vi "HEWH Standard MW100 Data.vi"(4 "Flow Selector":T1, 7 "Emerson Flow Meter Data Output":T2, 8 "Error In":errorcluster, 11 "MW100 Data Cluster":T3) -> (0 "Error Out":errorcluster, 2 "Hot Side Emerson Flow Meter Data":T2, 3 "Standard MW100 Data":string[][](array[string])=[["T1", "0.000"], ["T2", "0.000"], ["T3", "0.000"], ["T4", "0.000"], ["T5", "0.000"], ["T6", "0.000"], ["T7", "0.000"], ["T8", "0.000"], ["T9", "0.000"], ["T10", "0.000"], ["TC Tree Average", "0.000"], ["TC Down", "0.000"], ["RTD IN", "0.000"], ["RTD Out", "0.000"], ["RTD Ambient", "0.000"], ["Totalized Flow (Linear Link) - Calculated (Gallons)", "0.000"], ["Flow Rate (Linear Link) - Calculated (GPM)", "0.000"], ["Pressure - HI1", "0.000"], ["Pressure - HI2", "0.000"], ["Pressure - LOW", "0.000"], ["Pressure - PIN", "0.000"]])   [LabVIEW 2020]
uses:
  Type Definitions/HEWH MW100 Data Cluster.ctl
  Drivers/Emerson 5700 Transmitter/Type Definitions/Emerson 5700 Data.ctl
  Type Definitions/Flow Meter Selector.ctl
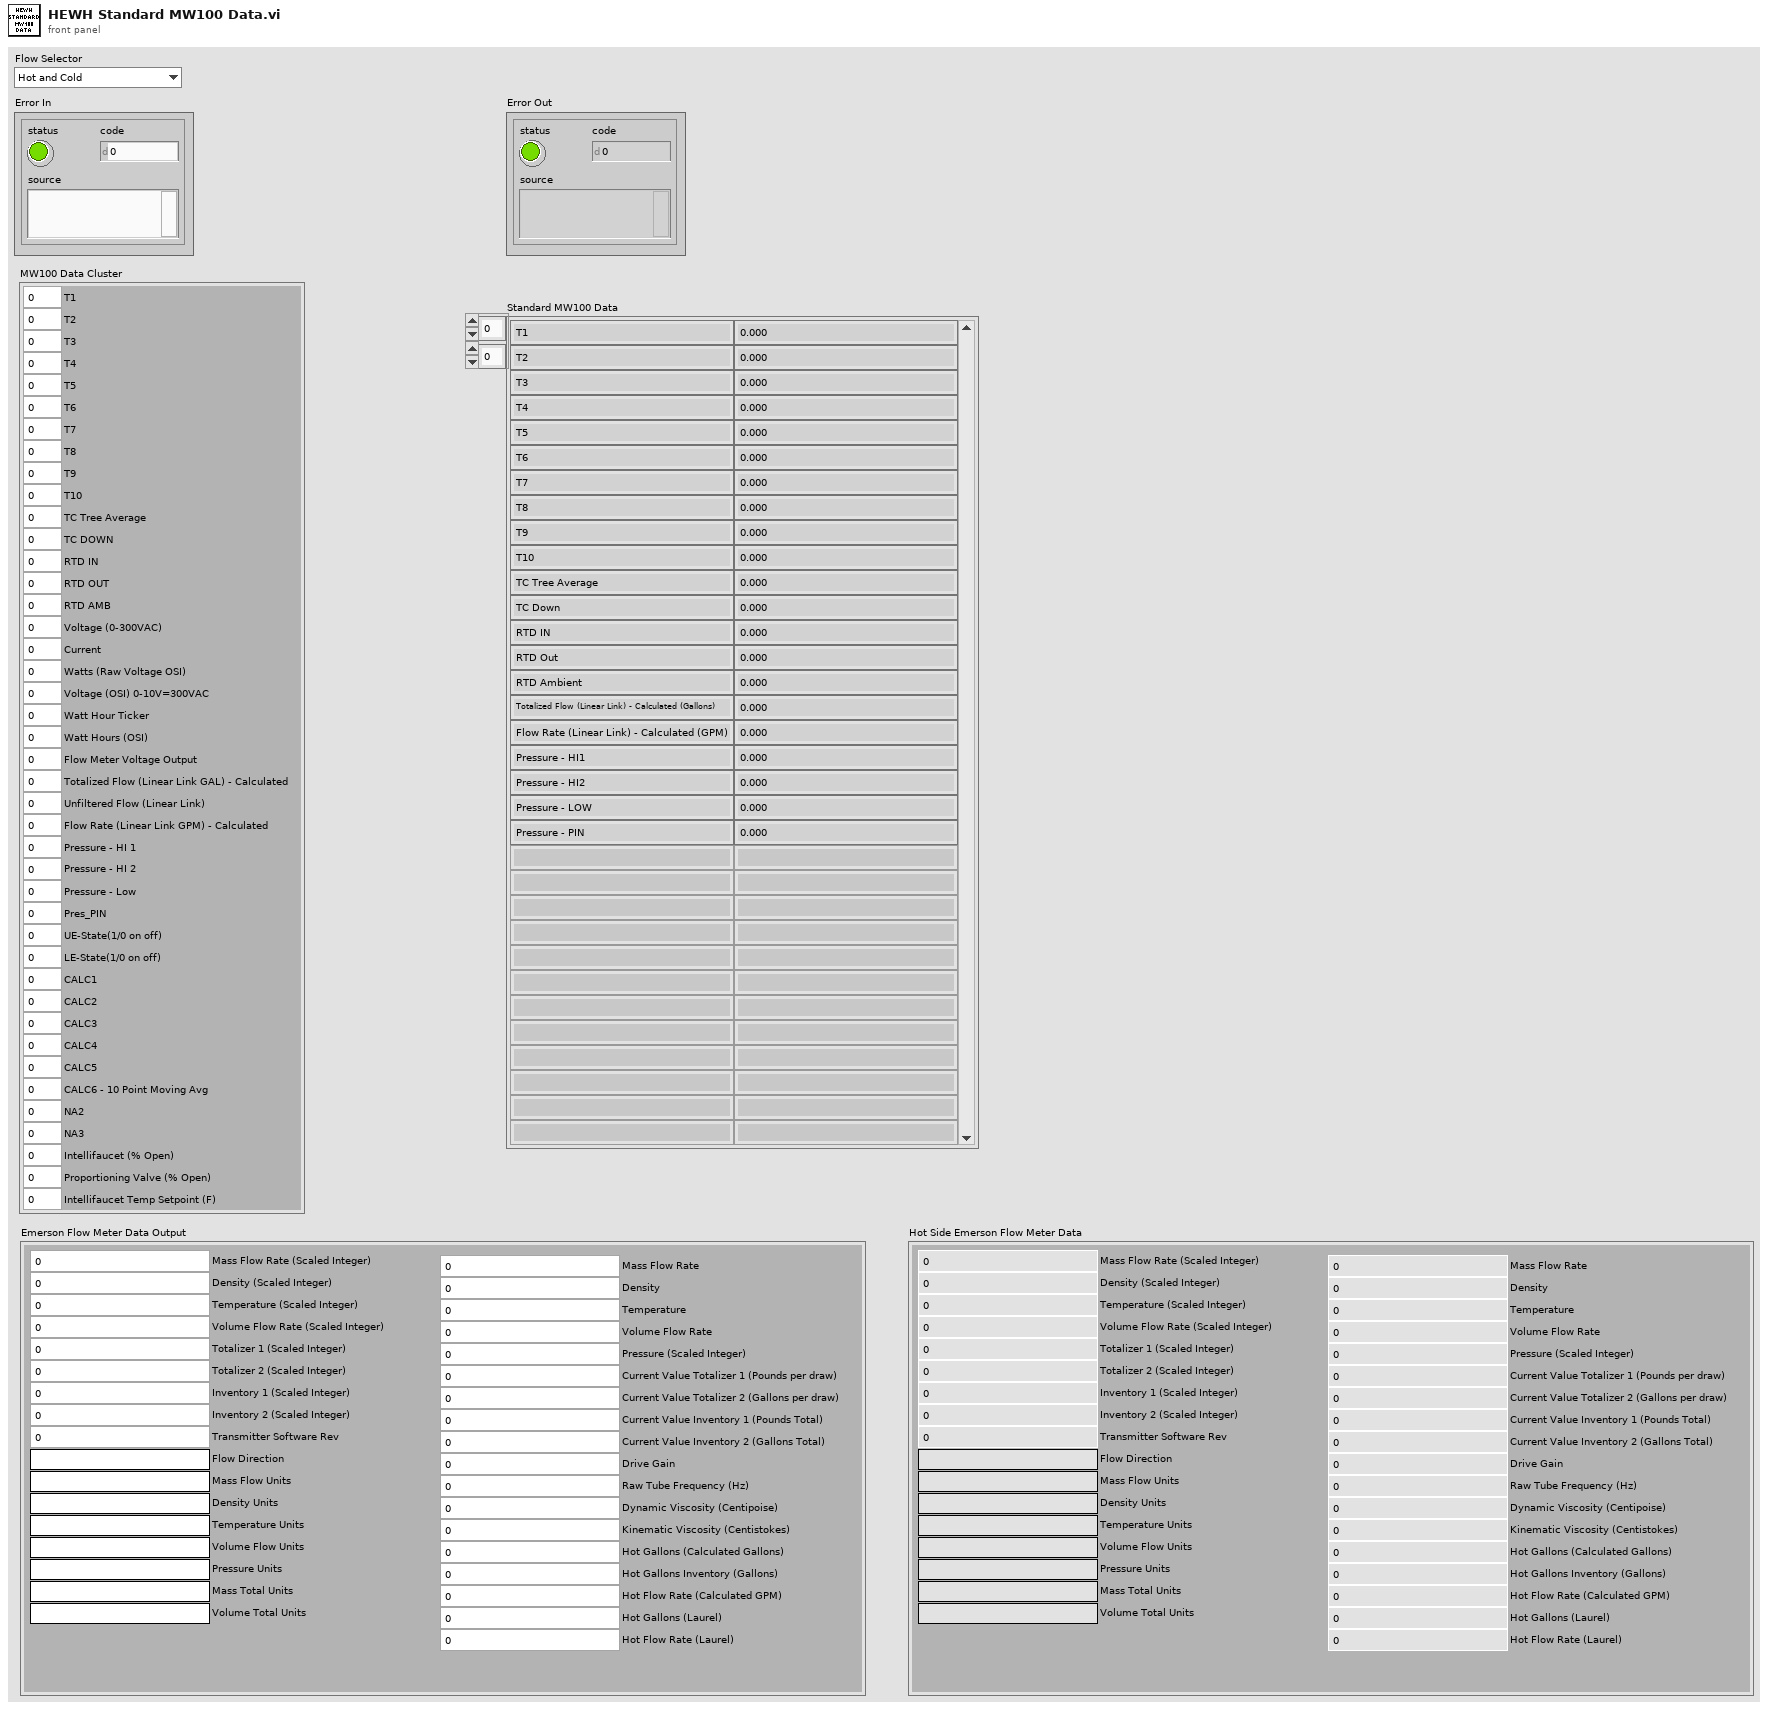
[diagram p1: front panel]
types:
  T1 = typedef "Flow Meter Selector.ctl" = enum16{"Hot and Cold", "Hot", "Cold", "None"}
  T2 = typedef "Emerson 5700 Data.ctl" = cluster{"Mass Flow Rate (Scaled Integer)":u16, "Density (Scaled Integer)":u16, "Temperature (Scaled Integer)":u16, "Volume Flow Rate (Scaled Integer)":u16, "Totalizer 1 (Scaled Integer)":u16, "Totalizer 2 (Scaled Integer)":u16, "Transmitter Software Rev":u16, "Flow Direction":string, "Mass Flow Units":string, "Density Units":string, "Temperature Units":string, "Volume Flow Units":string, "Pressure Units":string, "Mass Total Units":string, "Volume Total Units":string, "Inventory 1 (Scaled Integer)":u16, "Inventory 2 (Scaled Integer)":u16, "Mass Flow Rate":dbl, "Density":dbl, "Temperature":dbl, "Volume Flow Rate":dbl, "Pressure (Scaled Integer)":u16, "Current Value Totalizer 1 (Pounds per draw)":dbl, "Current Value Totalizer 2 (Gallons per draw)":dbl, "Current Value Inventory 1 (Pounds Total)":dbl, "Current Value Inventory 2 (Gallons Total)":dbl, "Drive Gain":dbl, "Raw Tube Frequency (Hz)":dbl, "Dynamic Viscosity (Centipoise)":dbl, "Kinematic Viscosity (Centistokes)":dbl, "Hot Gallons (Calculated Gallons)":dbl, "Hot Flow Rate (Calculated GPM)":dbl, "Hot Gallons Inventory (Gallons)":dbl, "Hot Flow Rate (Laurel)":dbl, "Hot Gallons (Laurel)":dbl}
  T3 = typedef "HEWH MW100 Data Cluster.ctl" = cluster{"T1":dbl, "T2":dbl, "T3":dbl, "T4":dbl, "T5":dbl, "T6":dbl, "T7":dbl, "T8":dbl, "T9":dbl, "T10":dbl, "TC Tree Average":dbl, "TC DOWN":dbl, "RTD IN":dbl, "RTD OUT":dbl, "RTD AMB":dbl, "Voltage (0-300VAC)":dbl, "Current":dbl, "Watts (Raw Voltage OSI)":dbl, "Voltage (OSI) 0-10V=300VAC":dbl, "Watt Hour Ticker":dbl, "Watt Hours (OSI)":dbl, "Flow Meter Voltage Output":dbl, "Totalized Flow (Linear Link GAL) - Calculated":dbl, "Unfiltered Flow (Linear Link)":dbl, "Flow Rate (Linear Link GPM) - Calculated":dbl, "Pressure - HI 1":dbl, "Pressure - HI 2":dbl, "Pressure - Low":dbl, "Pres_PIN":dbl, "UE-State(1/0 on off)":dbl, "LE-State(1/0 on off)":dbl, "CALC1":dbl, "CALC2":dbl, "CALC3":dbl, "CALC4":dbl, "CALC5":dbl, "CALC6 - 10 Point Moving Avg":dbl, "NA2":dbl, "NA3":dbl, "Intellifaucet (% Open)":dbl, "Proportioning Valve (% Open)":dbl, "Intellifaucet Temp Setpoint (F)":dbl}
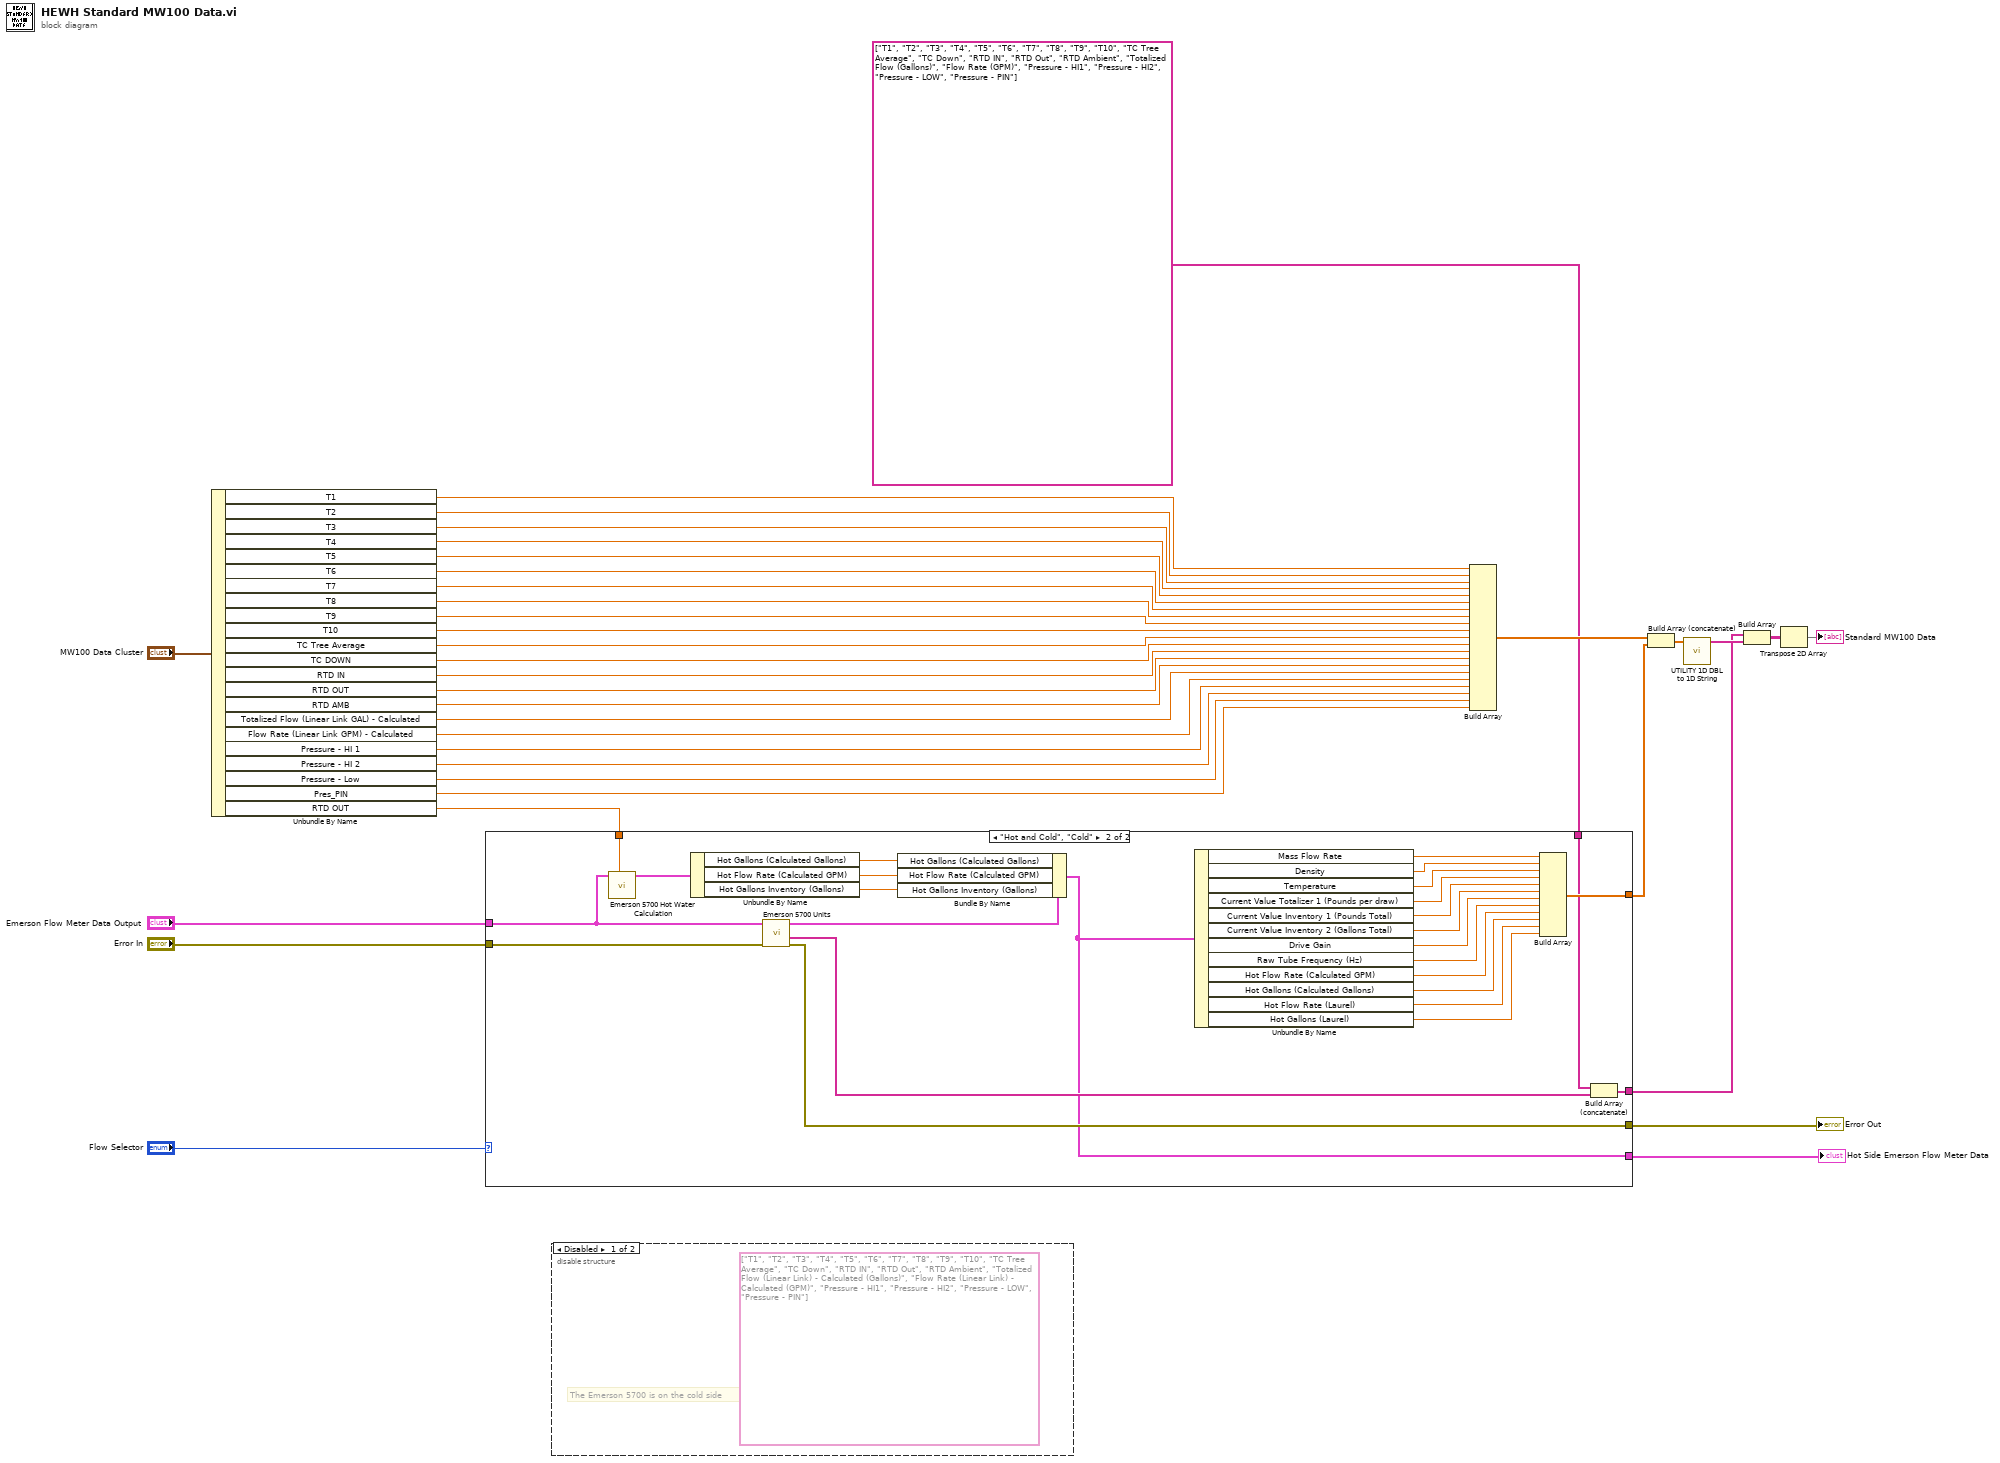
[diagram p0: block diagram]
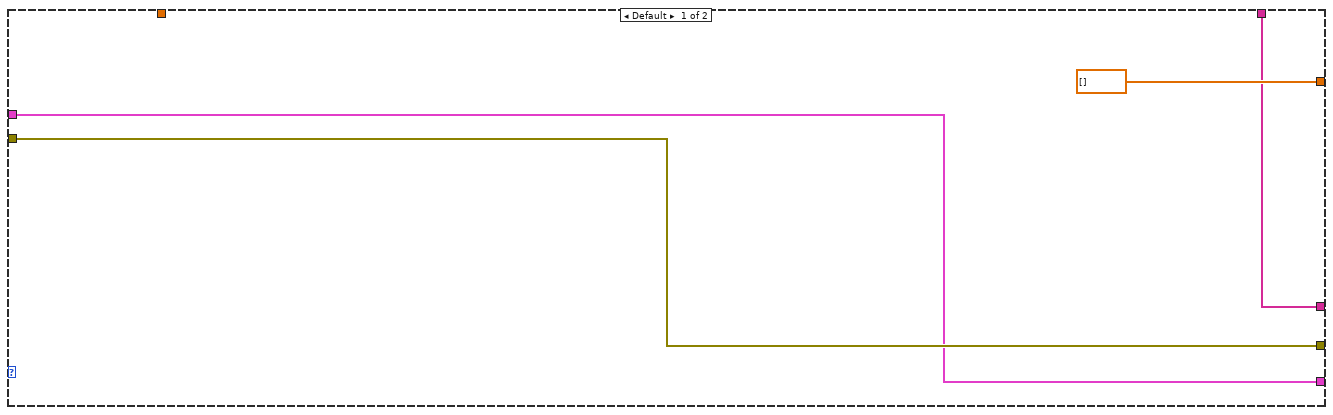
[diagram p3: hidden frame]
diagram:
  n1 = Unbundle By Name("MW100 Data Cluster") -> ("T1"=w18:dbl, "T2"=w19:dbl, "T3"=w20:dbl, "T4"=w21:dbl, "T5"=w22:dbl, "T6"=w23:dbl, "T7"=w24:dbl, "T8"=w25:dbl, "T9"=w26:dbl, "T10"=w27:dbl, "TC Tree Average"=w28:dbl, "TC DOWN"=w29:dbl, "RTD IN"=w30:dbl, "RTD OUT"=w31:dbl, "RTD AMB"=w32:dbl, "Totalized Flow (Linear Link GAL) - Calculated"=w13:dbl, "Flow Rate (Linear Link GPM) - Calculated"=w12:dbl, "Pressure - HI 1"=w33:dbl, "Pressure - HI 2"=w34:dbl, "Pressure - Low"=w35:dbl, "Pres_PIN"=w36:dbl, "RTD OUT"=w2:dbl)
  n2 = case shown="\"Hot and Cold\", \"Cold\"" "Flow Selector" {
    tunnel: [dbl[] [] w58] -> w10
    tunnel: string[] ["T1", "T2", "T3", "T4", "T5", "T6", "T7", "T8", "T9", "T10", "TC Tree Average", "TC Down", "RTD IN", "RTD Out", "RTD Ambient", "Totalized Flow (Gallons)", "Flow Rate (GPM)", "Pressure - HI1", "Pressure - HI2", "Pressure - LOW", "Pressure - PIN"] ("output array") -> [w39 w57]
    tunnel: [w39 w56] -> w7
    tunnel: "Error In" -> [w38 w51]
    tunnel: [w38 w53] -> w5
    tunnel: [w37 w41] -> w4
    tunnel: "Emerson Flow Meter Data Output" -> [w37 w50]
    tunnel: w2 -> [_ w49]
    frame Default {
    }
    frame "Hot and Cold", "Cold" {
      n3 = call "Emerson 5700 Hot Water Calculation.vi"("RTD Out (°F)"=w49, "Emerson Flow Meter Data Output"=w50) -> ("Emerson Flow Meter Data Output 2"=w48:T2)  [unwired: 8 in, 1 out]
      n4 = Unbundle By Name(w48) -> ("Hot Gallons (Calculated Gallons)"=w46:dbl, "Hot Flow Rate (Calculated GPM)"=w45:dbl, "Hot Gallons Inventory (Gallons)"=w44:dbl)
      n5 = call "Emerson 5700 Units.vi"("Error In"=w51, "Emerson Flow Meter Data Input"=w50) -> ("Error Out"=w53:errorcluster, "Basic Units"=w52:string[], "Emerson Flow Meter Data Output"=w47:T2)  [unwired: 6 in, 1 out]
      n6 = Bundle By Name(cluster=w47, "Hot Gallons (Calculated Gallons)"=w46, "Hot Flow Rate (Calculated GPM)"=w45, "Hot Gallons Inventory (Gallons)"=w44) -> (w41:T2)
      n7 = Unbundle By Name(w41) -> ("Mass Flow Rate"=w66:dbl, "Density"=w65:dbl, "Temperature"=w64:dbl, "Current Value Totalizer 1 (Pounds per draw)"=w63:dbl, "Current Value Inventory 1 (Pounds Total)"=w62:dbl, "Current Value Inventory 2 (Gallons Total)"=w61:dbl, "Drive Gain"=w60:dbl, "Raw Tube Frequency (Hz)"=w59:dbl, "Hot Flow Rate (Calculated GPM)"=w55:dbl, "Hot Gallons (Calculated Gallons)"=w54:dbl, "Hot Flow Rate (Laurel)"=w43:dbl, "Hot Gallons (Laurel)"=w42:dbl)
      n8 = Build Array(w66, w65, w64, w63, w62, w61, w60, w59, w55, w54, w43, w42) -> (w58:dbl[])
      n9 = Build Array (concatenate)(w57, w52) -> (w56:string[])
    }
  }
  "Error Out" <- w5
  "Hot Side Emerson Flow Meter Data" <- w4
  n10 = disable-structure shown="Disabled" {
    frame Disabled {
      (unwired) string[] ["T1", "T2", "T3", "T4", "T5", "T6", "T7", "T8", "T9", "T10", "TC Tree Average", "TC Down", "RTD IN", "RTD Out", "RTD Ambient", "Totalized Flow (Linear Link) - Calculated (Gallons)", "Flow Rate (Linear Link) - Calculated (GPM)", "Pressure - HI1", "Pressure - HI2", "Pressure - LOW", "Pressure - PIN"] ("output array")
      # "The Emerson 5700 is on the cold side"
    }
    frame Enabled {
    }
  }
  n11 = Build Array(w18, w19, w20, w21, w22, w23, w24, w25, w26, w27, w28, w29, w30, w31, w32, w13, w12, w33, w34, w35, w36) -> (w11:dbl[])
  n12 = Build Array (concatenate)(w11, w10) -> (w9:dbl[])
  n13 = call "UTILITY 1D DBL to 1D String.vi"("1D DBL"=w9) -> ("1D String"=w16:string[])  [unwired: 10 in]
  n14 = Build Array(w7, w16) -> (w17:string[][])
  n15 = Transpose 2D Array(2D array=w17) -> (transposed array=→"Standard MW100 Data":string[][])
